vi "readImageDataInImageTable.vi"(8 "error in":errorcluster, 11 "dataToQueryOfRead":T2) -> (0 "error out":errorcluster, 3 "ClusterFormat":T1)   [LabVIEW 2014]
uses:
  <vilib>/addons/database/Connection.llb/DB Tools Open Connec (String).vi
  <vilib>/addons/database/Auxilliary.llb/DB Tools Format Datetime String (Time Stamp).vi
  <vilib>/addons/database/NI_Database_API.lvlib
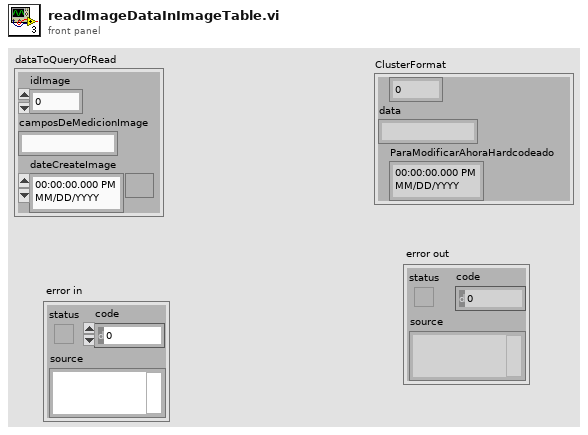
[diagram p1: front panel]
types:
  T1 = cluster{dbl, "data":string, "ParaModificarAhoraHardcodeado":timestamp}
  T2 = cluster{"idImage":dbl, "camposDeMedicionImage":string, "dateCreateImage":timestamp}
  T3 = typedef "NI_Database_API.lvlib/Conn ObjectReference.ctl" = refnum<k1>
  T4 = typedef "NI_Database_API.lvlib/DB Tools DataTypes.ctl" = enum16{"String", "Long (I32)", "Single (SGL)", "Double (DBL)", "Date/Time", "Binary"}
  T5 = cluster{"name":string, "database data type":T4, "defined size":i32}[]
  T6 = cluster{string, "camposDeMedicionImage":string, "date/time string":string}
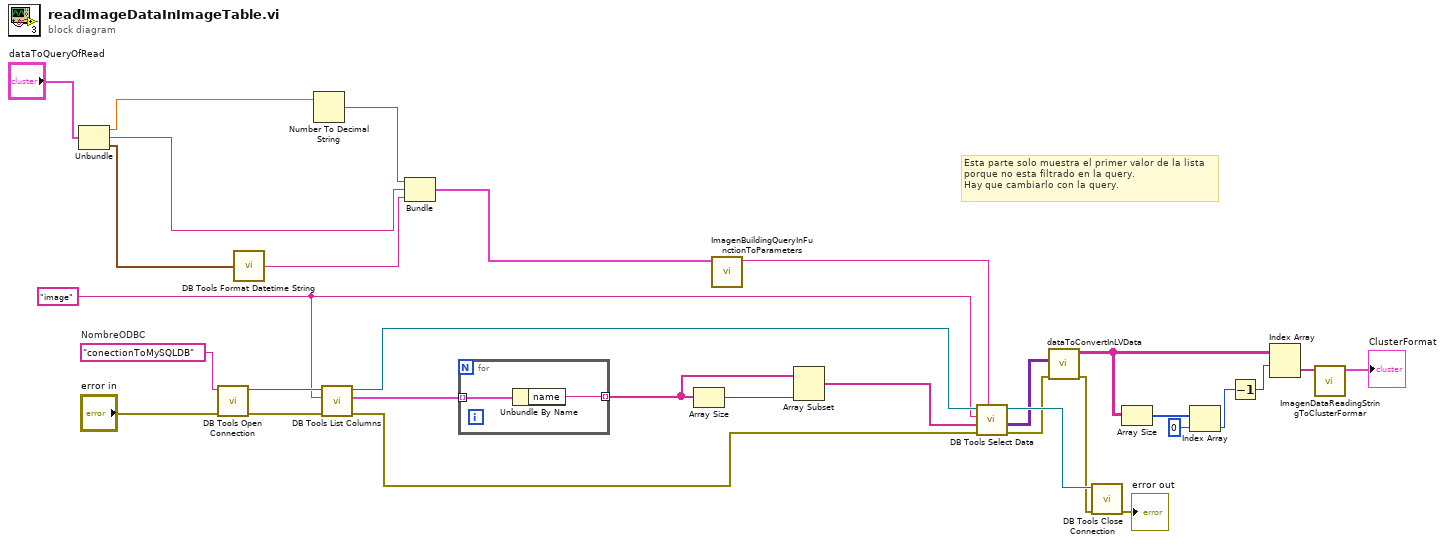
[diagram p0: block diagram]
diagram:
  w16 = "image" ("tableName")
  w31 = "conectionToMySQLDB"  # NombreODBC
  # "Esta parte solo muestra el primer valor de la lista\nporque no esta filtrado en la query.\nHay que cambiarlo con la query."
  n1 = Unbundle("dataToQueryOfRead") -> ("idImage"=w24:dbl, "camposDeMedicionImage"=w23:string, "dateCreateImage"=w22:timestamp)
  n2 = call-poly <vilib>:"DB Tools Open Connection.vi"("error in (no error)"="error in", "connection information"=w31) -> ("error out"=w29:errorcluster, "connection reference"=w30:T3)  [unwired: 6 in]
  n3 = call-poly <vilib>:"DB Tools Format Datetime String.vi"("time stamp"=w22) -> ("date/time string"=w25:string)
  n4 = Number To Decimal String(number=w24) -> (decimal integer string=w26:string)  [unwired: 1 in]
  n5 = call <vilib>:"DB Tools List Columns.vi"("error in (no error)"=w29, "table"=w16, "connection reference"=w30) -> ("error out"=w17:errorcluster, "column information"=w27:T5, "connection reference out"=w18:T3)  [unwired: 1 in, 1 out]
  n6 = Bundle(w26, "camposDeMedicionImage"=w23, "date/time string"=w25) -> (w15:T6)  [unwired: 1 in]
  n7 = for {
    tunnel: w27 -> [w33] mode=indexing
    tunnel: [w32] -> w20 mode=indexing
    n8 = Unbundle By Name(w33) -> ("name"=w32:string)
  }
  n9 = Array Size(array=w20) -> (size(s)=w21:i32)
  n10 = call "ImagenBuildingQueryInFunctionToParameters.vi"("ParameterToRead"=w15) -> ("QueryToRead"=w14:string)  [unwired: 10 in]
  n11 = Array Subset(array=w20, length=w21) -> (w19:string[])  [unwired: 1 in]
  n12 = call <vilib>:"DB Tools Select Data.vi"("condition"=w14, "error in (no error)"=w17, "columns"=w19, "table"=w16, "connection reference"=w18) -> ("error out"=w10:errorcluster, "data"=w11:variant[][], "connection reference out"=w13:T3)  [unwired: 1 in]
  n13 = call "dataToConvertInLVData.vi"("error in"=w10, "dataReadingIn"=w11) -> ("error out"=w9:errorcluster, "dataReadingOut"=w2:string[][])  [unwired: 8 in]
  n14 = call <vilib>:"DB Tools Close Connection.vi"("error in (no error)"=w9, "connection reference"=w13) -> ("error out"=→"error out":errorcluster)  [unwired: 5 in]
  n15 = Array Size(array=w2) -> (size(s)=w5:i32[])
  n16 = Index Array(array=w5, index=0) -> (element=w3:i32)
  n17 = Decrement(x=w3) -> (x-1=w1:i32)
  n18 = Index Array(array=w2, index (row)=w1) -> (element=w8:string[])  [unwired: 1 in]
  n19 = call "ImagenDataReadingStringToClusterFormar.vi"("StringFormat"=w8) -> ("ClusterFormat"=→"ClusterFormat":T2)  [unwired: 10 in]
